vi "Read Timeout.vi"(8 "error in (no error)":errorcluster, 11 "WriteCommand in":refnum<class "WriteCommand.lvclass">) -> (0 "error out":errorcluster, 2 "Timeout":u32=2000 min=1 step=1, 3 "WriteCommand out":refnum<class "WriteCommand.lvclass">)   [LabVIEW 2023, in "HAF.lvlib" / "WriteCommand.lvclass"]
doc: "Returns the current Timeout. If zero, returns 5000 (milliseconds.)"
uses:
  WriteCommand.lvclass
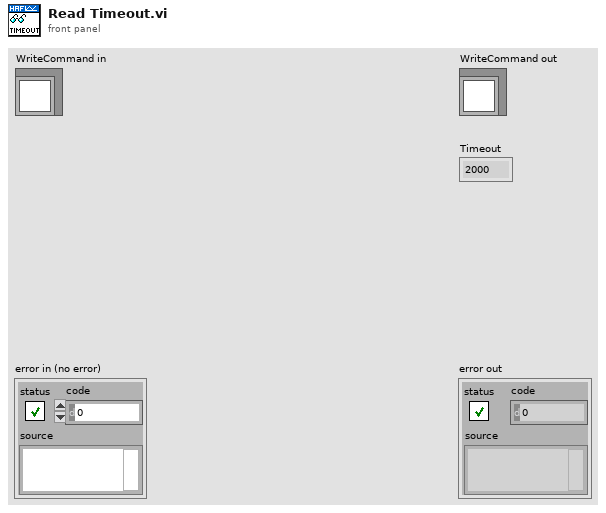
[diagram p1: front panel]
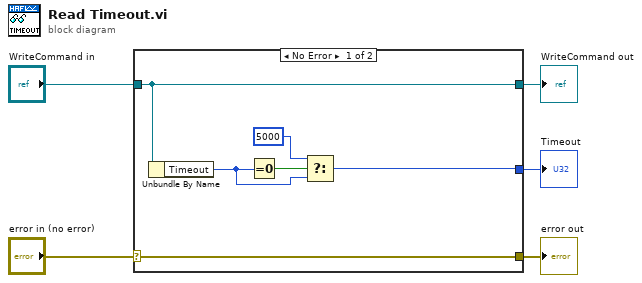
[diagram p0: block diagram]
diagram:
  n1 = case shown="No Error" "error in (no error)" {
    selector: "error in (no error)" -> [w11 w12]
    tunnel: [w11 w12] -> w4
    tunnel: [w10 w13] -> w2
    tunnel: "WriteCommand in" -> [w10 w13]
    tunnel: [w6 _] -> w1
    frame No Error {
      n2 = Unbundle By Name(w10) -> ("Timeout"=w8:u32)
      n3 = Equal To 0?(x=w8) -> (x = 0?=w9:bool)
      n4 = Select(t=u32 5000, s=w9, f=w8) -> (s? t:f=w6:u32)
    }
    frame Error {
    }
  }
  "error out" <- w4
  "WriteCommand out" <- w2
  "Timeout" <- w1
